vi "PDF Creation.vi"() -> ()   [LabVIEW 2020]
uses:
  C:/Users/Simon/Documents/GitHub/LV-WebView2/Source/Libs/Microsoft.Web.WebView2.WinForms.dll
  Libs/Microsoft.Web.WebView2.WinForms.dll
  C:/Users/Simon/Documents/GitHub/LV-WebView2/Source/Libs/Microsoft.Web.WebView2.Core.dll
  Libs/Microsoft.Web.WebView2.Core.dll
  Webview2 Lib/WebView2 Control Object/Read Print Options.vi
  Webview2 Lib/WebView2 Control Object/WebView2 Control.lvclass
panel:
  in  "WebView2":refnum<k24>(container)
  in  "stop":bool
  out "Timeout":bool
  in  "PDF":bool
  in  "String":string
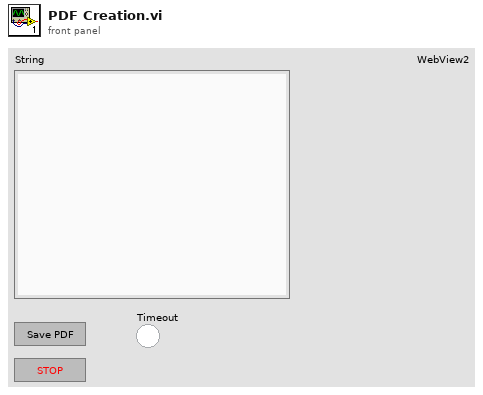
[diagram p1: front panel]
types:
  T1 = cluster{"search string":string, "replace string (\"\")":string}[]
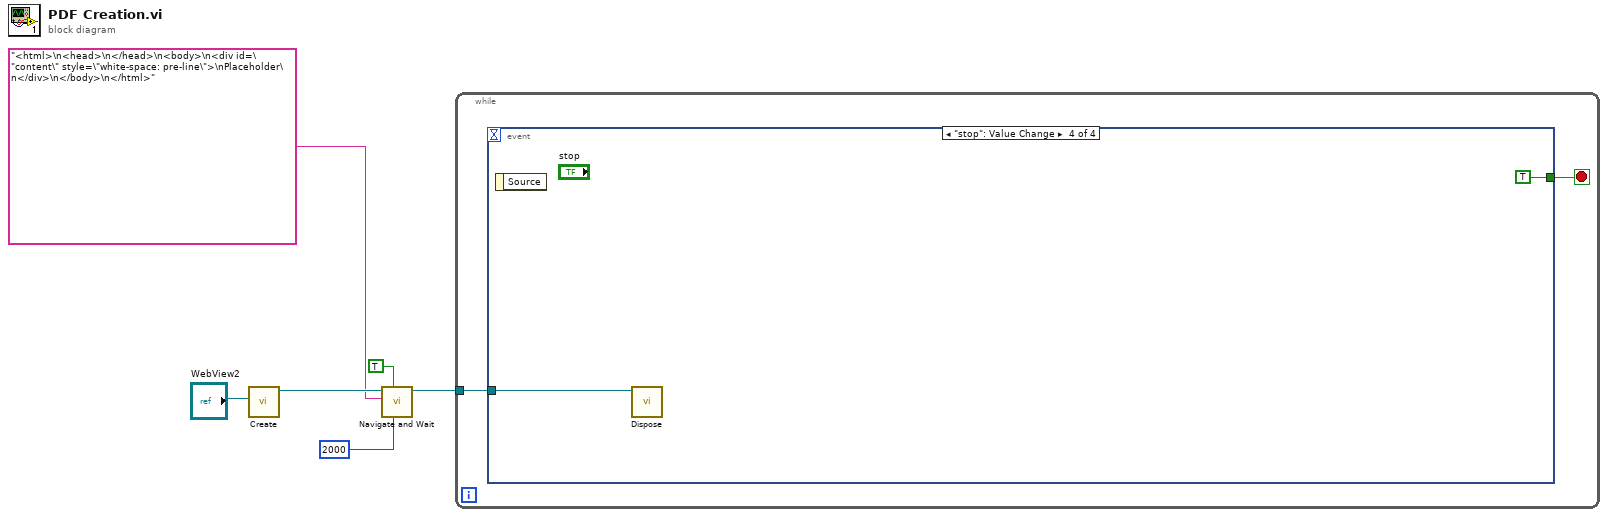
[diagram p0: block diagram]
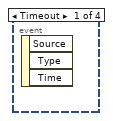
[diagram p2: hidden frame]
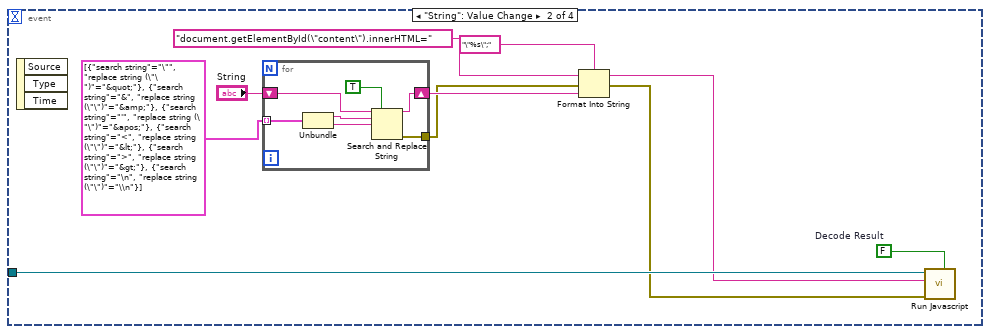
[diagram p3: hidden frame]
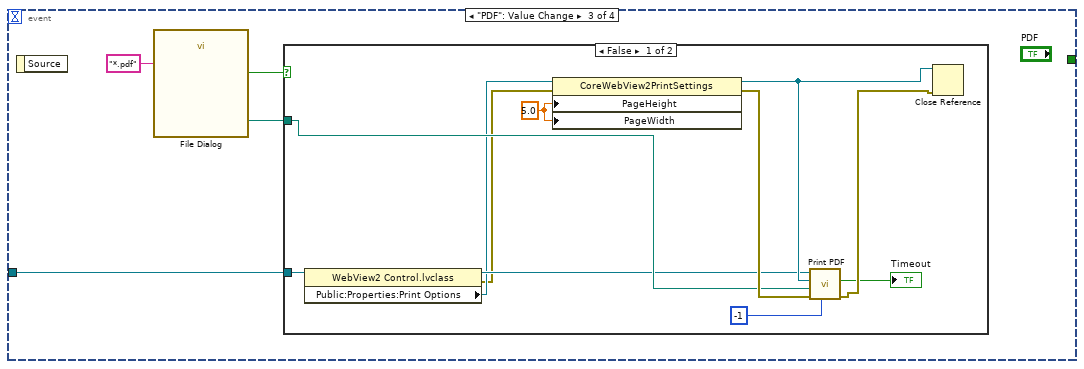
[diagram p4: hidden frame]
diagram:
  n1 = call "Create.vi"("WebView2 Control"="WebView2") -> ("WebView2 Control out"=w5:refnum<class "WebView2 Control.lvclass">)  [unwired: 9 in, 1 out]
  n2 = call "Navigate and Wait.vi"("Timeout (Inf)"=2000, "html Source (URL)"=TRUE, "Source"="<html>\n<head>\n</head>\n<body>\n<div id=\"content\" style=\"white-space: pre-line\">\nPlaceholder\n</div>\n</body>\n</html>", "WebView2 Control in"=w5) -> ("WebView2 Control out"=w1:refnum<class "WebView2 Control.lvclass">)  [unwired: 5 in, 2 out]
  n3 = while {
    tunnel: w1 -> [w7]
    stop <- w8 stop-if-true
    n4 = event shown="[3] \"stop\": Value Change" {
      selector: _ -> [_ _ _ _]
      dyn-events: _ -> [_ _ _ _]
      timeout: _ -> [_ _ _ _]
      tunnel: [_ _ _ TRUE] -> w8
      tunnel: w7 -> [_ w12 w26 w41]
      event Timeout {
        n5 = event-data() -> ()  [unwired: 1 in, 3 out]
      }
      event "String": Value Change {
        w9 = FALSE  # Decode Result
        n6 = event-data() -> ()  [unwired: 1 in, 3 out]
        n7 = for {
          tunnel: [w22] -> w14
          shift-right: [w24] -> w15
          shift-left: "String" -> [w25]
          tunnel: T1 [{"search string"="\"", "replace string (\"\")"="&quot;"}, {"search string"="&", "replace string (\"\")"="&amp;"}, {"search string"="'", "replace string (\"\")"="&apos;"}, {"search string"="<", "replace string (\"\")"="&lt;"}, {"search string"=">", "replace string (\"\")"="&gt;"}, {"search string"="\n", "replace string (\"\")"="\\n"}] -> [w21] mode=indexing
          n8 = Unbundle(w21) -> ("search string"=w20:string, "replace string (\"\")"=w19:string)
          n9 = Search and Replace String(replace all?=TRUE ("replace all? (F)"), input string=w25, search string=w20, replace string=w19) -> (result string=w24:string, error out=w22:errorcluster)  [unwired: 4 in, 2 out]
        }
        n10 = Format Into String(format string="\"%s\";", initial string="document.getElementById(\"content\").innerHTML=" ("javaScript"), error in=w14, w15) -> (resulting string=w11:string, error out=w10:errorcluster)
        n11 = call "Run Javascript.vi"("Decode Result (T)"=w9, "error in (no error)"=w10, "javaScript"=w11, "WebView2 Control in"=w12) -> ()  [unwired: 5 in, 3 out]
      }
      event "PDF": Value Change {
        n12 = event-data() -> ()  [unwired: 1 in, 1 out]
        n13 = call "File Dialog"("pattern (all files)"="*.pdf") -> ("selected path"=w28:path, "cancelled"=w27:bool)  [unwired: 11 in, 2 out]
        n14 = case shown="False" w27 {
          tunnel: w28 -> [w34 _]
          tunnel: w26 -> [w39 _]
          frame False {
            w40 = 5.0 ("PageHeight")
            n15 = property class="WebView2 Control.lvclass"(reference=w39) -> (reference out=w33:refnum<class "WebView2 Control.lvclass">, error out=w31:errorcluster, "Public:Properties:Print Options"=w32:refnum<k24>)  [unwired: 1 in]
            n16 = property class="CoreWebView2PrintSettings"(reference=w32, error in=w31, "PageHeight"=w40, "PageWidth"=w40) -> (reference out=w38:refnum<k24>, error out=w36:errorcluster)
            n17 = call "Print PDF.vi"("Timeout ms"=-1, "error in (no error)"=w36, "PDF File Path"=w34, "printSettings"=w38, "WebView2 Control in"=w33) -> ("error out"=w37:errorcluster, "Timeout"=→"Timeout":bool)  [unwired: 4 in, 1 out]
            n18 = Close Reference(reference=w38, error in (no error)=w37) -> ()  [unwired: 1 out]
          }
          frame True {
          }
        }
      }
      event "stop": Value Change {
        n19 = event-data() -> ()  [unwired: 1 in, 1 out]
        n20 = call "Dispose.vi"("WebView2 Control in"=w41) -> ()  [unwired: 10 in, 1 out]
      }
    }
  }
